vi "Software Timing (on Demand).vi"() -> ()   [LabVIEW 2015]
uses:
  <vilib>/DAQmx/create/channels.llb/DAQmx Create Channel (DI-Digital Input).vi
  <vilib>/DAQmx/read.llb/DAQmx Read (Digital 1D Bool 1Chan 1Samp).vi
panel:
  in  "Loop Wait Time":u32(slide) scale=0.0..1000.0
  in  "stop":bool
  out "data":bool[](array[boolean])
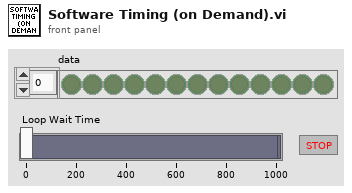
[diagram p1: front panel]
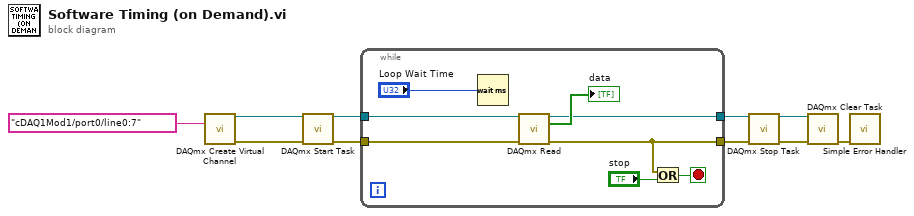
[diagram p0: block diagram]
diagram:
  n1 = call-poly <vilib>:"DAQmx Create Virtual Channel.vi"("lines"=tag "cDAQ1Mod1/port0/line0:7") -> ("task out"=w9:refnum<k21>, "error out"=w8:errorcluster)  [unwired: 13 in]
  n2 = call <vilib>:"DAQmx Start Task.vi"("task/channels in"=w9, "error in"=w8) -> ("task out"=w7:refnum<k21>, "error out"=w6:errorcluster)  [unwired: 12 in]
  n3 = while {
    tunnel: w7 -> [w18]
    tunnel: w6 -> [w17]
    tunnel: [w13] -> w4
    tunnel: [w12] -> w2
    stop <- w14 stop-if-true
    n4 = Wait (ms)(milliseconds to wait="Loop Wait Time") -> ()  [unwired: 1 out]
    n5 = call-poly <vilib>:"DAQmx Read.vi"("task/channels in"=w18, "error in"=w17) -> ("task out"=w13:refnum<k21>, "data"=→"data":bool[], "error out"=w12:errorcluster)  [unwired: 11 in]
    n6 = Or(x=w12, y="stop") -> (x .or. y?=w14:bool)
  }
  n7 = call <vilib>:"DAQmx Stop Task.vi"("task/channels in"=w4, "error in"=w2) -> ("task out"=w5:refnum<k21>, "error out"=w3:errorcluster)  [unwired: 12 in]
  n8 = call <vilib>:"DAQmx Clear Task.vi"("task in"=w5, "error in"=w3) -> ("error out"=w1:errorcluster)  [unwired: 13 in]
  n9 = call <vilib>:"Simple Error Handler.vi"("error in (no error)"=w1) -> ()  [unwired: 4 in, 5 out]
